vi "App Global.vi"(7 "Mode":T1, 9 "CPU Usage:":dbl=7.74131899555212 format="%.1f", 10 "Login":bool, 11 "Client?":bool) -> (1 "CPU Usage OUT":dbl, 2 "Login OUT":bool, 3 "Client? OUT":bool)   [LabVIEW 2019]
uses:
  Controls/App Global Mode.ctl
panel:
  in  "Login":bool
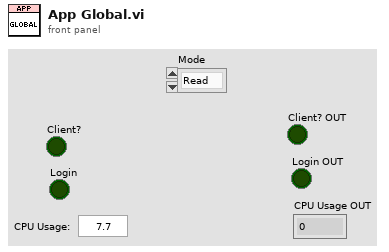
[diagram p1: front panel]
types:
  T1 = typedef "App Global Mode.ctl" = enum16{"Read", "Write Client", "Write Login"}
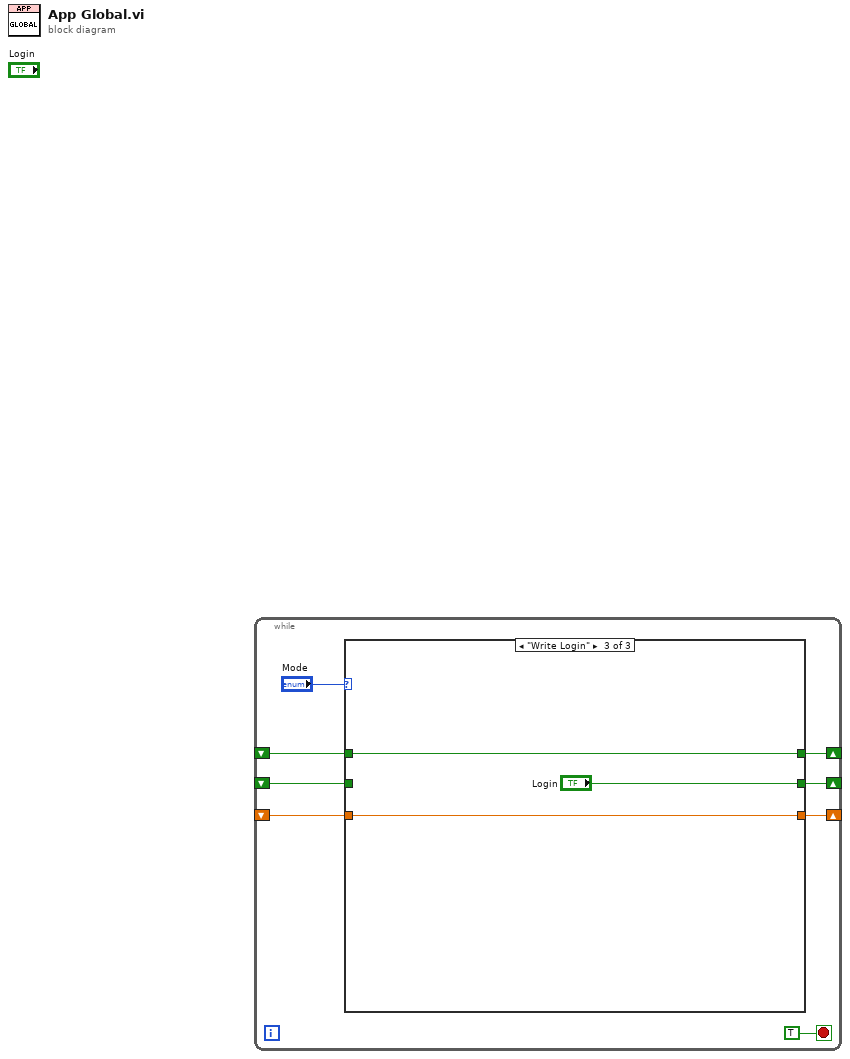
[diagram p0: block diagram]
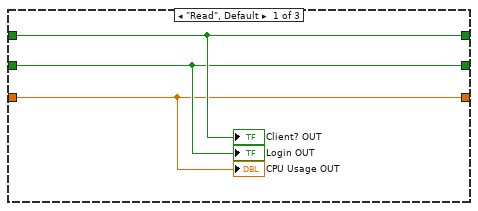
[diagram p2: hidden frame]
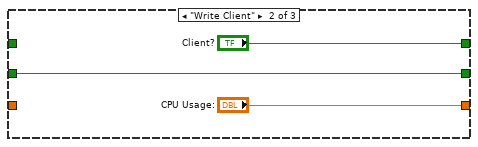
[diagram p3: hidden frame]
diagram:
  n1 = while {
    shift-right: [w7] -> _
    shift-left: _ -> [w4]
    shift-right: [w6] -> _
    shift-left: _ -> [w3]
    shift-right: [w5] -> _
    shift-left: _ -> [w2]
    stop <- TRUE stop-if-true
    n2 = case shown="\"Write Login\"" "Mode" {
      tunnel: [w11 "Client?" w17] -> w7
      tunnel: [w10 w12 "Login"] -> w6
      tunnel: [w9 "CPU Usage:" w16] -> w5
      tunnel: w4 -> [w11 _ w17]
      tunnel: w3 -> [w10 w12 _]
      tunnel: w2 -> [w9 _ w16]
      frame "Read", Default {
        "Client? OUT" <- w11
        "Login OUT" <- w10
        "CPU Usage OUT" <- w9
      }
      frame "Write Client" {
      }
      frame "Write Login" {
      }
    }
  }
